vi "Get Teams from User.vi"(6 "Authorization":T2[](array[typedef]), 8 "error in (no error)":errorcluster, 11 "User GID":string) -> (0 "error out":errorcluster, 3 "Teams Out":T1(array[cluster]))   [LabVIEW 2016]
uses:
  <vilib>/addons/_JKI.lib/REST Client/classes/REST Client/HTTP Header.ctl
  <vilib>/addons/_JKI.lib/REST Client/classes/REST Client/REST Client.lvclass
  <vilib>/addons/_JKI.lib/Serialization/JSON/JKI JSON Serialization.lvlib
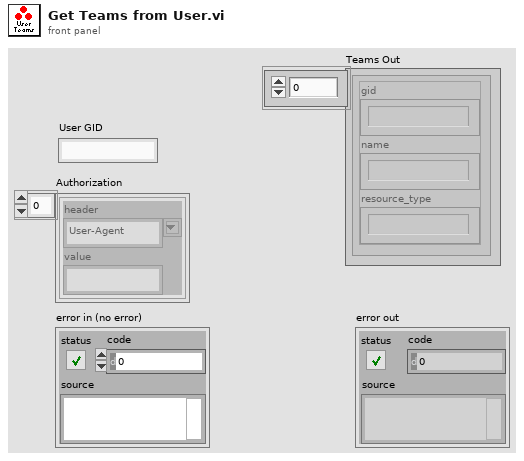
[diagram p1: front panel]
types:
  T1 = cluster{"gid":string, "name":string, "resource_type":string}[]
  T2 = typedef "REST Client.lvlib/REST Client.lvclass/HTTP Header.ctl" = cluster{"header":string, "value":string}
  T3 = cluster{"data":cluster{"gid":string, "name":string, "resource_type":string}[]}
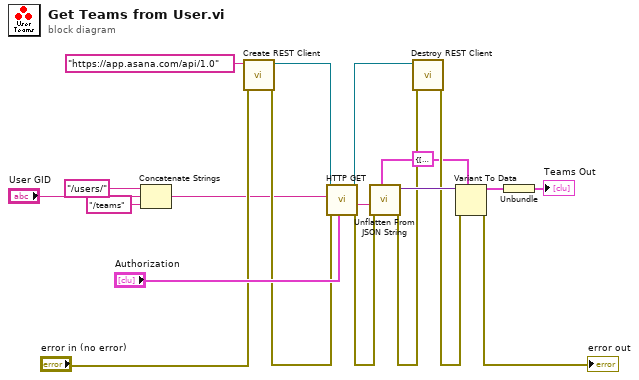
[diagram p0: block diagram]
diagram:
  w7 = T3 {"data"=[{"gid"="", "name"="", "resource_type"=""}, {"gid"="", "name"="", "resource_type"=""}]}
  n1 = Concatenate Strings("/users/", "User GID", "/teams" ("string")) -> (w2:string)
  n2 = call <vilib>:"Create REST Client.vi"("error in (no error)"="error in (no error)", "Base URL"="https://app.asana.com/api/1.0") -> ("error out"=w14:errorcluster, "REST Client out"=w17:refnum<class "REST Client.lvclass">)  [unwired: 8 in]
  n3 = call-dynamic "HTTP GET.vi"("request specific headers"="Authorization", "error in (no error)"=w14, "Path"=w2, "REST Client in"=w17) -> ("error out"=w11:errorcluster, "Response body"=w12:string, "REST Client out"=w16:refnum<class "REST Client.lvclass">)  [unwired: 2 in, 3 out]
  n4 = call <vilib>:"Unflatten From JSON String.vi"("Type and Defaults"=w7, "error in (no error)"=w11, "JSON String"=w12) -> ("error out"=w10:errorcluster, "Variant"=w13:variant)  [unwired: 7 in]
  n5 = call-dynamic "Destroy REST Client.vi"("error in (no error)"=w10, "REST Client in"=w16) -> ("error out"=w9:errorcluster)  [unwired: 9 in]
  n6 = Variant To Data(error in=w9, type=w7, Variant=w13) -> (data=w6:T3, error out=→"error out":errorcluster)
  n7 = Unbundle(w6) -> ("data"=→"Teams Out":T1)
